vi "SaveAnalogueStatsforEachBlock.vi"() -> (5 "Plug in titles":string[](array[string]), 7 "Plug in values":string[](array[string]))   [LabVIEW 2018]
uses:
  Globals/Meas_global.vi
  <vilib>/Analysis/NI_AALBase.lvlib
panel:
  out "Table":string[][](table)
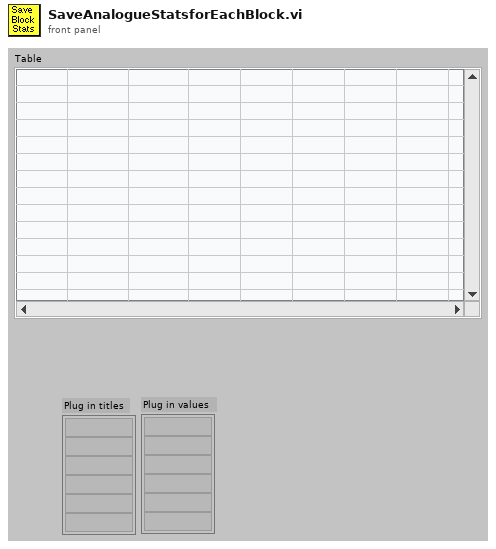
[diagram p1: front panel]
types:
  T1 = typedef "Analysis_info_cluster.ctl" = cluster{"Colour":u32, "Inst type":T2, "Inst name":string, "Symbol":string, "Code name":string, "Extra Info":string, "Inst Array":T3, "Extra Titles":string[], "Extra Values":string[], "U":dbl, "u^2":dbl, "u^3":dbl, "u^4":dbl, "Skew_u":dbl, "Kurt_u":dbl, "Sd Error in Mean":dbl, "% u'/U":dbl, "X":dbl, "Y":dbl, "Z":dbl, "Timescale integral Estimate":dbl, "Sd Error in Variance":dbl, "Calib File":path, "Calib Constants":dbl[], "Output Position":bool, "Stats":enum16{"None", "Basic", "Full"}, "Av Sampling Rate":dbl, "Av No of Samples":dbl, "Total Meas Time (s)":dbl, "ADAM Ch Name":string, "Max value":dbl, "Min value":dbl, "Req Sample Rate Hz":dbl, "Sync Delay Time (s)":dbl, "Ch No":i16, "Device":string, "Use Latest Calib":bool, "Port":string, "Metadata Ch Names":string[], "Metadata Ch Values":string[]}
  T2 = typedef "Inst_type.ctl" = enum16{"Propeller anemometer", "Raw voltage", "Pressure Transducer", "Pitot-static tube", "Preston tube", "Hot wire", "Cross wire 1", "Cross wire 2", "Generic Linear", "Generic Polynomial", "Generic BackPoly", "Fast FID", "Thermocouple", "Cold wire", "Pulsed Wire", "LDA Vel", "LDA Tran time", "LDA Arr time", "Microphone"}
  T3 = typedef "Instrument_Array.ctl" = enum16{"PWA", "LDA", "Analogue"}
  T4 = typedef "Time_Trace_Cluster.ctl" = cluster{"Weighting":dbl[], "Time (s)":dbl[], "Voltage":dbl[], "Eng Values":dbl[]}
  T5 = enum16{"Save no data", "Save data in new files", "Save data in existing files"}
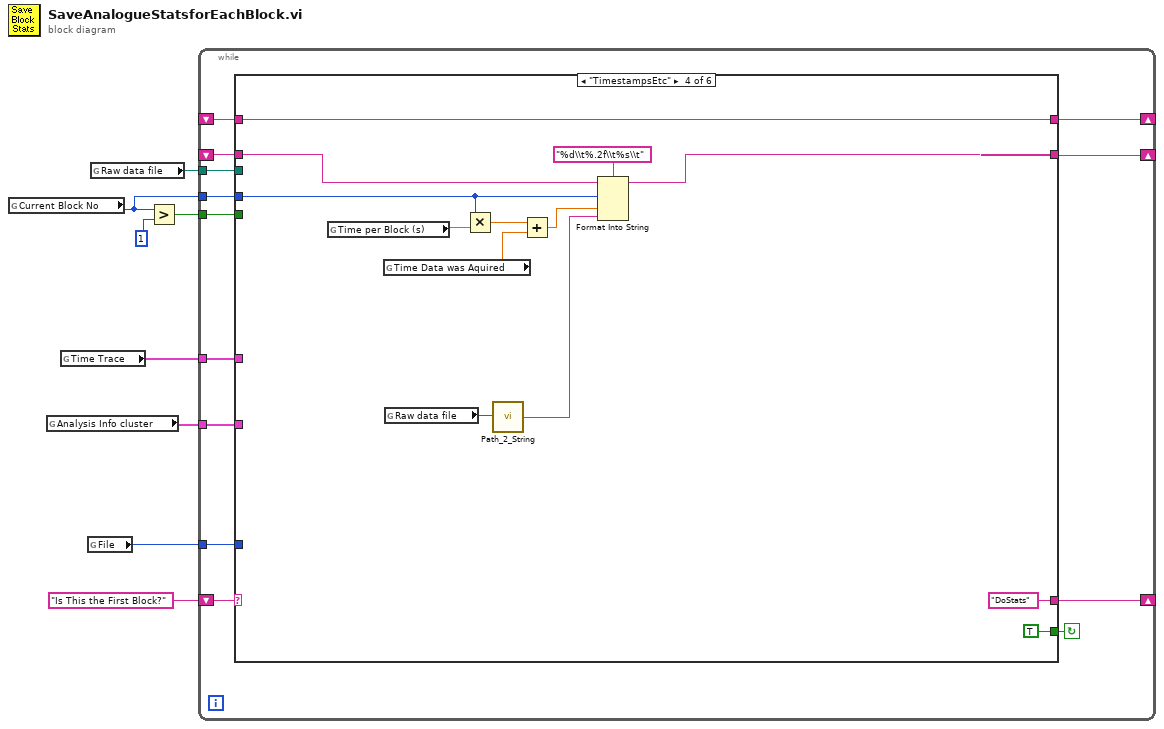
[diagram p0: block diagram]
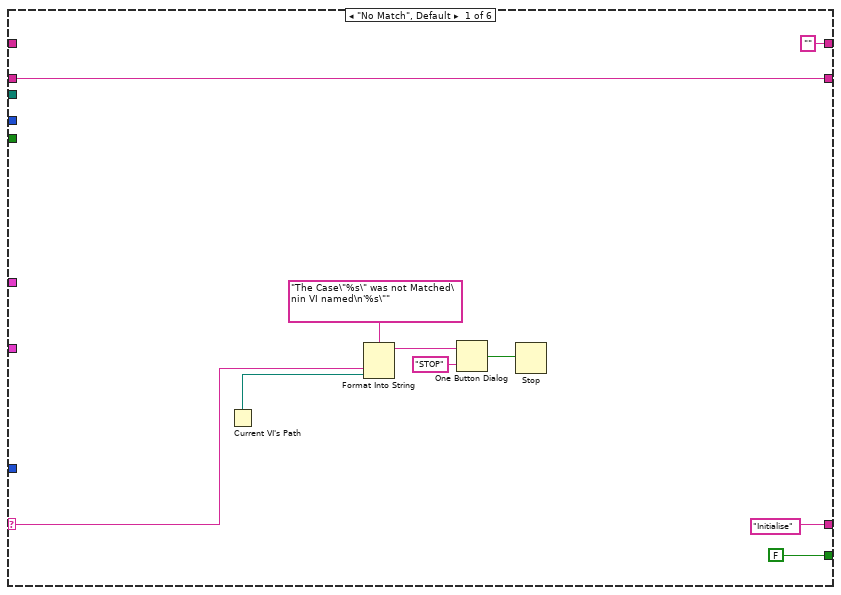
[diagram p2: hidden frame]
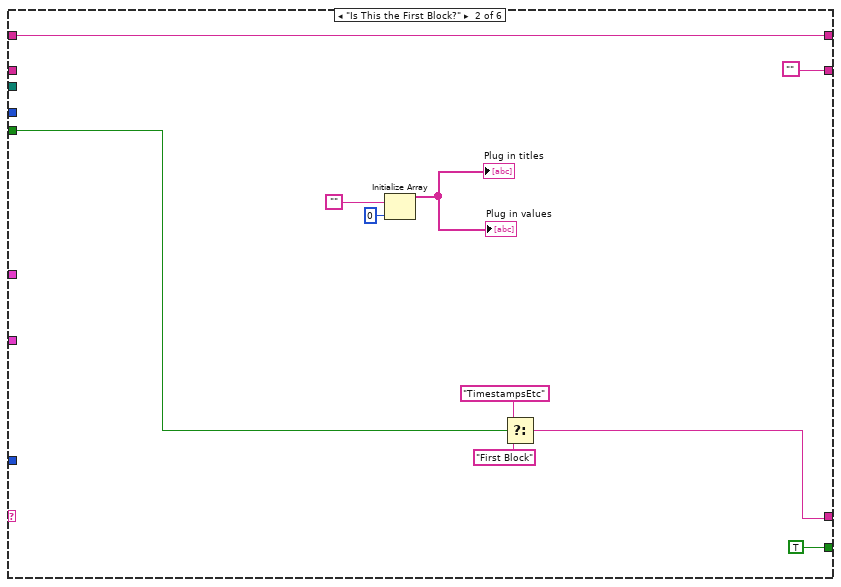
[diagram p3: hidden frame]
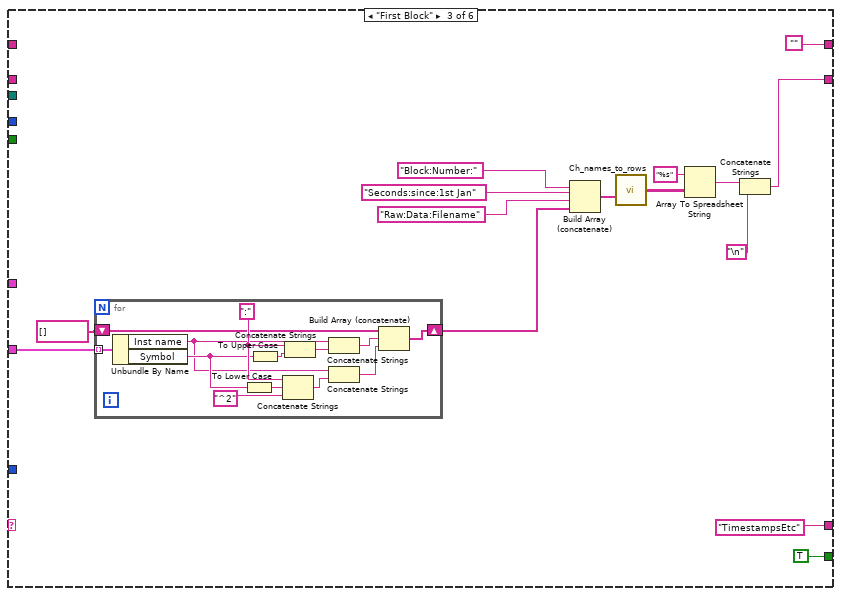
[diagram p4: hidden frame]
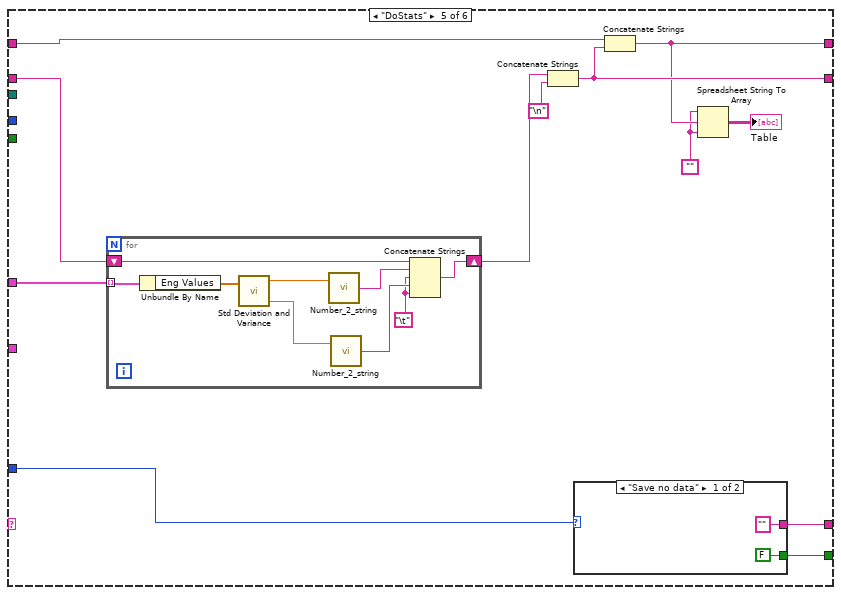
[diagram p5: hidden frame]
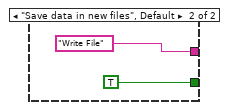
[diagram p6: hidden frame]
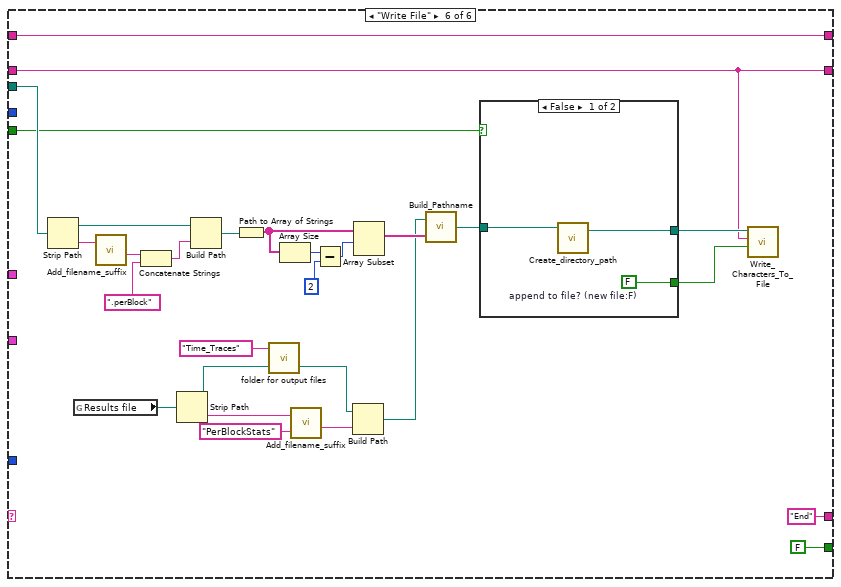
[diagram p7: hidden frame]
diagram:
  n1 = global read "Meas_global.vi" "Current Block No"() -> (w2:i32)
  n2 = global read "Meas_global.vi" "Analysis Info cluster"() -> (w4:T1[])
  n3 = global read "Meas_global.vi" "Time Trace"() -> (w3:T4[])
  n4 = global read "Meas_global.vi" "File"() -> (w1:T5)
  n5 = global read "Meas_global.vi" "Raw data file"() -> (w7:path)
  n6 = Greater?(x=w2, y=1) -> (0:w5:bool)
  n7 = while {
    shift-left: "Is This the First Block?" -> [w19]
    shift-right: [w20] -> _
    shift-right: [w12] -> _
    shift-left: _ -> [w17]
    tunnel: w7 -> [w18]
    tunnel: w5 -> [w16]
    tunnel: w4 -> [w15]
    tunnel: w3 -> [w14]
    tunnel: w2 -> [w13]
    shift-right: [w10] -> _
    shift-left: _ -> [w11]
    tunnel: w1 -> [w9]
    stop <- w21 continue-if-true
    n8 = case shown="\"TimestampsEtc\"" w19 {
      selector: w19 -> [w23 _ _ _ _ _]
      tunnel: [FALSE TRUE TRUE TRUE w94 FALSE] -> w21
      tunnel: ["Initialise" w37 "TimestampsEtc" ("t") "DoStats" ("t") w93 "End" ("t")] -> w20
      tunnel: w18 -> [_ _ _ _ _ w131]
      tunnel: [w24 "" w46 w77 w90 w117] -> w12
      tunnel: w17 -> [w24 _ _ w78 w83 w117]
      tunnel: w16 -> [_ w38 _ _ _ w128]
      tunnel: w15 -> [_ _ w49 _ _ _]
      tunnel: w14 -> [_ _ _ _ w92 _]
      tunnel: w13 -> [_ _ _ w70 _ _]
      tunnel: w11 -> [_ w34 _ w79 w89 w116]
      tunnel: ["" w34 "" w79 w88 w116] -> w10
      tunnel: w9 -> [_ _ _ _ w87 _]
      frame "No Match", Default {
        n9 = Current VI's Path() -> (path=w26:path)
        n10 = Format Into String(format string="The Case\"%s\" was not Matched\nin VI named\n'%s\"" ("Format String"), w23, w26) -> (resulting string=w29:string)  [unwired: 2 in, 1 out]
        n11 = One Button Dialog(message=w29, button name ("OK")="STOP") -> (true=w27:bool)
        n12 = Stop(stop? (T)=w27) -> ()
      }
      frame "Is This the First Block?" {
        n13 = Initialize Array("", 0) -> (→"Plug in values" →"Plug in titles":string[])
        n14 = Select(t="TimestampsEtc", s=w38, f="First Block") -> (s? t:f=w37:string)
      }
      frame "First Block" {
        n15 = for {
          shift-right: [w58] -> w43
          shift-left: string[] [] -> [w61]
          tunnel: w49 -> [w57] mode=indexing
          w66 = ":" ("string")
          n16 = Unbundle By Name(w57) -> ("Inst name"=w62:string, "Symbol"=w64:string)
          n17 = To Lower Case(string=w64) -> (all lower case string=w65:string)
          n18 = To Upper Case(1:w64) -> (0:w63:string)
          n19 = Concatenate Strings(w66, w65, "^2") -> (w68:string)
          n20 = Concatenate Strings(w66, w63) -> (w67:string)
          n21 = Concatenate Strings(w62, w67) -> (w60:string)
          n22 = Concatenate Strings(w62, w68) -> (w59:string)
          n23 = Build Array (concatenate)(w61, w60, w59) -> (w58:string[])
        }
        n24 = Build Array (concatenate)("Block:Number:", "Seconds:since:1st Jan", "Raw:Data:Filename", w43) -> (w51:string[])
        n25 = call "Ch_names_to_rows.vi"("Channel Names"=w51) -> ("3 Row names"=w50:string[][])
        n26 = Array To Spreadsheet String(array=w50, 3:"%s" ("format string")) -> (spreadsheet string=w48:string)  [unwired: 1 out]
        n27 = Concatenate Strings(w48, "\n") -> (w46:string)
      }
      frame "TimestampsEtc" {
        n28 = global read "Meas_global.vi" "Time per Block (s)"() -> (w71:dbl)
        n29 = global read "Meas_global.vi" "Time Data was Aquired"() -> (w75:dbl)
        n30 = global read "Meas_global.vi" "Raw data file"() -> (w76:path)
        n31 = Multiply(x=w70, y=w71) -> (x*y=w72:dbl)
        n32 = call "Path_2_String.vi"("Real Path"=w76) -> ("Path String"=w74:string)
        n33 = Add(x=w72, y=w75) -> (x+y=w73:dbl)
        n34 = Format Into String(format string="%d\\t%.2f\\t%s\\t", initial string=w78, w70, w73, w74) -> (resulting string=w77:string)  [unwired: 1 in, 1 out]
      }
      frame "DoStats" {
        w85 = ""
        n35 = for {
          tunnel: w92 -> [w105] mode=indexing
          shift-right: [w107] -> w91
          shift-left: w83 -> [w106]
          w99 = "\t"
          n36 = Unbundle By Name(w105) -> ("Eng Values"=w100:dbl[])
          n37 = call <vilib>:"Std Deviation and Variance.vi"("X"=w100) -> ("mean"=w104:dbl, "variance"=w103:dbl)  [unwired: 1 in, 1 out]
          n38 = call "Number_2_string.vi"("number"=w104) -> ("String"=w101:string)  [unwired: 1 in]
          n39 = call "Number_2_string.vi"("number"=w103) -> ("String"=w102:string)  [unwired: 1 in]
          n40 = Concatenate Strings(w106, w101, w99, w102, w99) -> (w107:string)
        }
        n41 = Concatenate Strings(w91, "\n") -> (w90:string)
        n42 = case shown="\"Save no data\"" w87 {
          tunnel: [FALSE TRUE] -> w94
          tunnel: ["" "Write File"] -> w93
          frame "Save no data" {
          }
          frame "Save data in new files", Default {
          }
        }
        n43 = Concatenate Strings(w89, w90) -> (w88:string)
        n44 = Spreadsheet String To Array(format string=w85, spreadsheet string=w88, array type (2D Dbl)=w85) -> (array=→"Table":string[][])  [unwired: 1 in]
      }
      frame "Write File" {
        n45 = Strip Path(path=w131) -> (stripped path=w133:path, name=w119:string)
        n46 = global read "Meas_global.vi" "Results file"() -> (w115:path)
        n47 = call "Add_filename_suffix.vi"("Filename"=w119) -> ("Base name"=w118:string)  [unwired: 1 in, 3 out]
        n48 = Concatenate Strings(w118, ".perBlock" ("Substring")) -> (w134:string)
        n49 = Strip Path(path=w115) -> (stripped path=w112:path, name=w114:string)
        n50 = Build Path(base path=w133, name or relative path=w134) -> (appended path=w132:path)
        n51 = Path to Array of Strings(0:w132) -> (2:w125:string[])  [unwired: 1 out]
        n52 = call "folder for output files.vi"("results folder"=w112, "folder name"="Time_Traces" ("name or relative path")) -> ("appended path"=w111:path)  [unwired: 1 out]
        n53 = Array Size(array=w125) -> (size(s)=w124:i32)
        n54 = call "Add_filename_suffix.vi"("Filename"=w114, "Suffix to add"="PerBlockStats") -> ("Base name"=w113:string)  [unwired: 3 out]
        n55 = Subtract(x=w124, y=2) -> (x-y=w122:i32)
        n56 = Build Path(base path=w111, name or relative path=w113) -> (appended path=w108:path)
        n57 = Array Subset(array=w125, index=w122) -> (w121:string[])  [unwired: 1 in]
        n58 = call "Build_Pathname.vi"("PathElements"=w121, "PathnameIn"=w108) -> ("AppendedPath"=w120:path)
        n59 = case shown="False" w128 {
          tunnel: [w138 w140] -> w130
          tunnel: w120 -> [w137 w139]
          tunnel: [w136 w139] -> w129
          frame False {
            w138 = FALSE  # append to file? (new file:F)
            n60 = call "Create_directory_path.vi"("Path name"=w137) -> ("Path name Out"=w136:path)  [unwired: 2 in, 1 out]
          }
          frame True {
            w140 = TRUE  # append to file? (new file:F)
          }
        }
        n61 = call "Write_Characters_To_File.vi"("file path (dialog if empty)"=w129, "character string"=w117, "append to file? (new file:F)"=w130) -> ()  [unwired: 2 in, 4 out]
      }
    }
  }
